vi "sub_SDR_mimo_MuxPorts.vi"(3 "Port 2 in":cdb[](array[numeric]), 5 "Port 1 in":cdb[](array[numeric])) -> (1 "Out":cdb[][](array[numeric]))   [LabVIEW 2012]
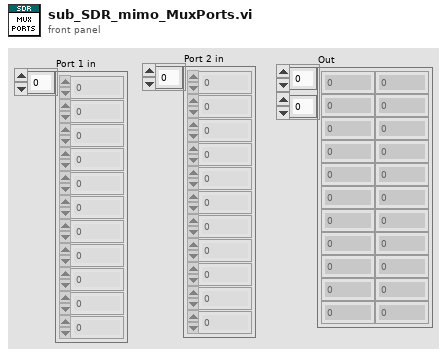
[diagram p1: front panel]
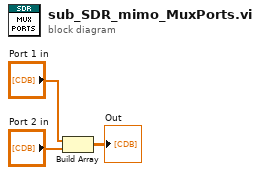
[diagram p0: block diagram]
diagram:
  n1 = Build Array("Port 1 in", "Port 2 in") -> (→"Out":cdb[][])
